vi "SSC DCPower Configure Output Connected.vi"(0 "DCPower SSC in":T1[](array[typedef]), 5 "Output Connected":bool, 11 "error in":errorcluster) -> (4 "DCPower SSC out":T1[](array[typedef]), 15 "error out":errorcluster)   [LabVIEW 2020]
doc: "This VI configures output enabled on the channels."
uses:
  SSC DCPower.ctl
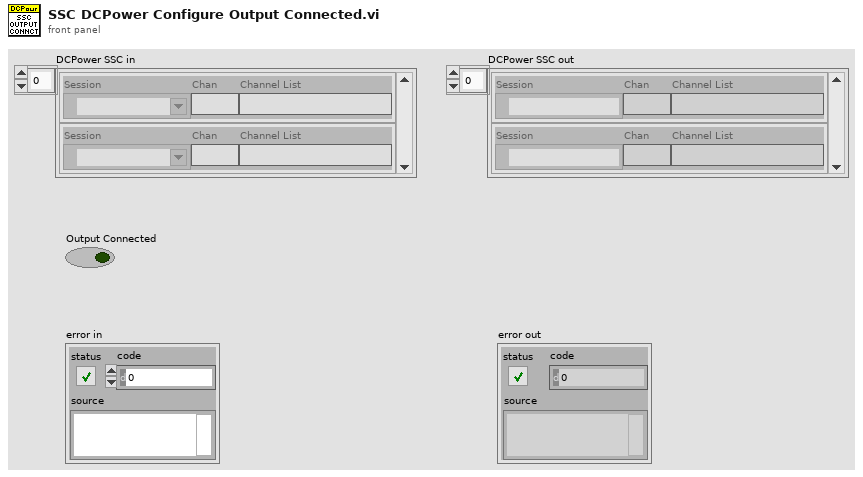
[diagram p1: front panel]
types:
  T1 = typedef "SSC DCPower.ctl" = cluster{"Session":refnum<k15>, "Chan":string, "Channel List":string}
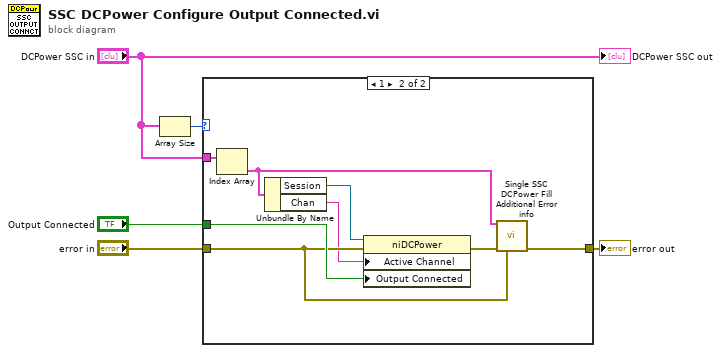
[diagram p0: block diagram]
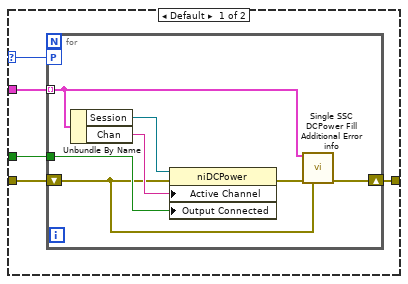
[diagram p2: hidden frame]
diagram:
  n1 = Array Size(array="DCPower SSC in") -> (size(s)=w2:i32)
  n2 = case shown="1" w2 {
    selector: w2 -> [w7 _]
    tunnel: [w10 w25] -> w5
    tunnel: "Output Connected" -> [w9 w24]
    tunnel: "error in" -> [w8 w23]
    tunnel: "DCPower SSC in" -> [w6 w22]
    frame Default {
      n3 = for {
        tunnel: w6 -> [w12] mode=indexing
        tunnel: w9 -> [w16]
        workers-P: w7 -> [_]
        shift-right: [w13] -> w10
        shift-left: w8 -> [w11]
        n4 = Unbundle By Name(w12) -> ("Session"=w15:refnum<k15>, "Chan"=w14:string)
        n5 = property class="niDCPower"(reference=w15, error in=w11, "Active Channel"=w14, "Output Connected"=w16) -> (error out=w17:errorcluster)  [unwired: 1 out]
        n6 = call "Single SSC DCPower Fill Additional Error info.vi"("DCPower SSC in"=w12, "error in"=w17, "previous error in"=w11) -> ("error out"=w13:errorcluster)  [unwired: 12 in]
      }
    }
    frame 1 {
      n7 = Index Array(array=w22) -> (element=w18:T1)  [unwired: 1 in]
      n8 = Unbundle By Name(w18) -> ("Session"=w20:refnum<k15>, "Chan"=w19:string)
      n9 = property class="niDCPower"(reference=w20, error in=w23, "Active Channel"=w19, "Output Connected"=w24) -> (error out=w21:errorcluster)  [unwired: 1 out]
      n10 = call "Single SSC DCPower Fill Additional Error info.vi"("DCPower SSC in"=w18, "error in"=w21, "previous error in"=w23) -> ("error out"=w25:errorcluster)  [unwired: 12 in]
    }
  }
  "error out" <- w5
  "DCPower SSC out" <- "DCPower SSC in"
